vi "BT Tx Test Get Default LSL.vi"(8 "error in (no error)":errorcluster, 11 "Template Tx Test in":refnum<class "niDTS BT Tx Test.lvclass">) -> (0 "error out":errorcluster, 2 "Default LSL":T1 {"OBW Resutls"."Stop Frequency (Hz)" format="%#_4p"; "OBW Resutls"."Start Frequency (Hz)" format="%#_4p"}, 3 "Template Tx Test out":refnum<class "niDTS BT Tx Test.lvclass">)   [LabVIEW 2015, in "niDTS BT.lvlib" / "niDTS BT Tx Test.lvclass"]
uses:
  niDTS BT Tx Test.lvclass
  Includes/niDTS BT Tx Test INC Results.ctl
  Includes/niDTS BT Tx Test INC IBE Results.ctl
  Includes/niDTS BT Tx Test INC OBW Results.ctl
  Includes/niDTS BT Tx Test INC TXP Results.ctl
  Includes/niDTS BT Tx Test INC DEVM Results.ctl
  Includes/niDTS BT Tx Test INC CF Stability Results.ctl
  Includes/niDTS BT Tx Test INC CFO Resutls.ctl
  Includes/niDTS BT Tx Test INC Character Results.ctl
  niDTS BT Tx Test.lvclass/niDTS BT Tx Test.ctl
  Includes/niDTS BT Tx Test INC Default Limits.vi
  niDTS BT.lvlib
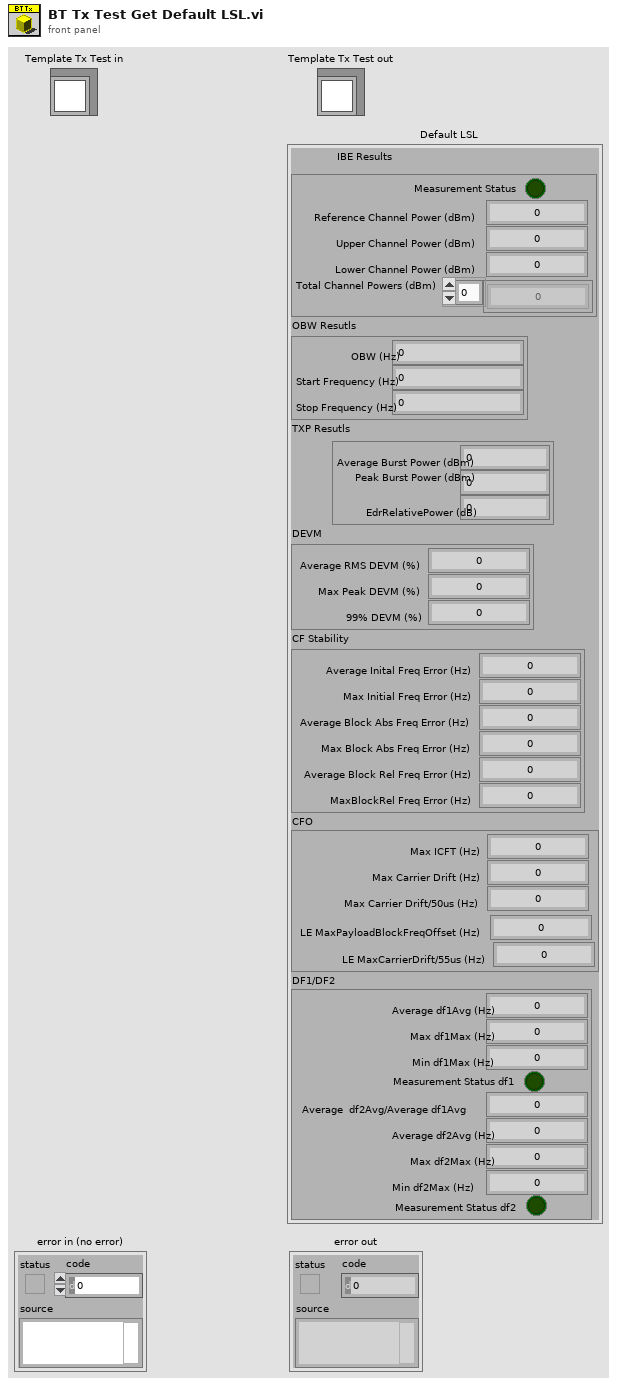
[diagram p1: front panel]
types:
  T1 = typedef "niDTS BT.lvlib/niDTS BT Tx Test INC Results.ctl" = cluster{"IBE Results":T2, "OBW Resutls":T3, "TXP Resutls":T4, "DEVM":T5, "CF Stability":T6, "CFO":T7, "DF1/DF2":T8}
  T2 = typedef "niDTS BT.lvlib/niDTS BT Tx Test INC IBE Results.ctl" = cluster{"Measurement Status":bool, "Reference Channel Power (dBm)":dbl, "Upper Channel Power (dBm)":dbl, "Lower Channel Power (dBm)":dbl, "Total Channel Powers (dBm)":dbl[]}
  T3 = typedef "niDTS BT.lvlib/niDTS BT Tx Test INC OBW Results.ctl" = cluster{"OBW (Hz)":dbl, "Start Frequency (Hz)":dbl, "Stop Frequency (Hz)":dbl}
  T4 = typedef "niDTS BT.lvlib/niDTS BT Tx Test INC TXP Results.ctl" = cluster{"Average Burst Power (dBm)":dbl, "Peak Burst Power (dBm)":dbl, "EdrRelativePower (dB)":dbl}
  T5 = typedef "niDTS BT.lvlib/niDTS BT Tx Test INC DEVM Results.ctl" = cluster{"Average RMS DEVM (%)":dbl, "Max Peak DEVM (%)":dbl, "99% DEVM (%)":dbl}
  T6 = typedef "niDTS BT.lvlib/niDTS BT Tx Test INC CF Stability Results.ctl" = cluster{"Average Inital Freq Error (Hz)":dbl, "Max Initial Freq Error (Hz)":dbl, "Average Block Abs Freq Error (Hz)":dbl, "Max Block Abs Freq Error (Hz)":dbl, "Average Block Rel Freq Error (Hz)":dbl, "MaxBlockRel Freq Error (Hz)":dbl}
  T7 = typedef "niDTS BT.lvlib/niDTS BT Tx Test INC CFO Resutls.ctl" = cluster{"Max ICFT (Hz)":dbl, "Max Carrier Drift (Hz)":dbl, "Max Carrier Drift/50us (Hz)":dbl, "LE MaxPayloadBlockFreqOffset (Hz)":dbl, "LE MaxCarrierDrift/55us (Hz)":dbl}
  T8 = typedef "niDTS BT.lvlib/niDTS BT Tx Test INC Character Results.ctl" = cluster{"Average df1Avg (Hz)":dbl, "Max df1Max (Hz)":dbl, "Min df1Max (Hz)":dbl, "Measurement Status df1":bool, "Average  df2Avg/Average df1Avg":dbl, "Average df2Avg (Hz)":dbl, "Max df2Max (Hz)":dbl, "Min df2Max (Hz)":dbl, "Measurement Status df2":bool}
  T9 = typedef "niDTS BT.lvlib/niDTS BT INC Packet Type.ctl" = enum16{"NULL", "POLL", "FHS", "DM1", "DH1", "HV1", "HV2", "HV3", "EV3", "DV", "AUX1", "DM3", "DH3", "EV4", "EV5", "DM5", "DH5", "LE-TP"}
  T10 = typedef "niDTS BT.lvlib/niDTS BT INC Standard.ctl" = enum16{"BDR", "EDR", "LE-TP"}
  T11 = typedef "niDTS BT.lvlib/niDTS BT Tx Test INC BD Payload Data.ctl" = enum16{"0", "1", "01", "00001111", "PN9", "AUTO"}
  T12 = typedef "niDTS BT.lvlib/niDTS BT Tx Test INC Modulation Characteristics.ctl" = enum16{"DF1", "DF2", "BOTH"}
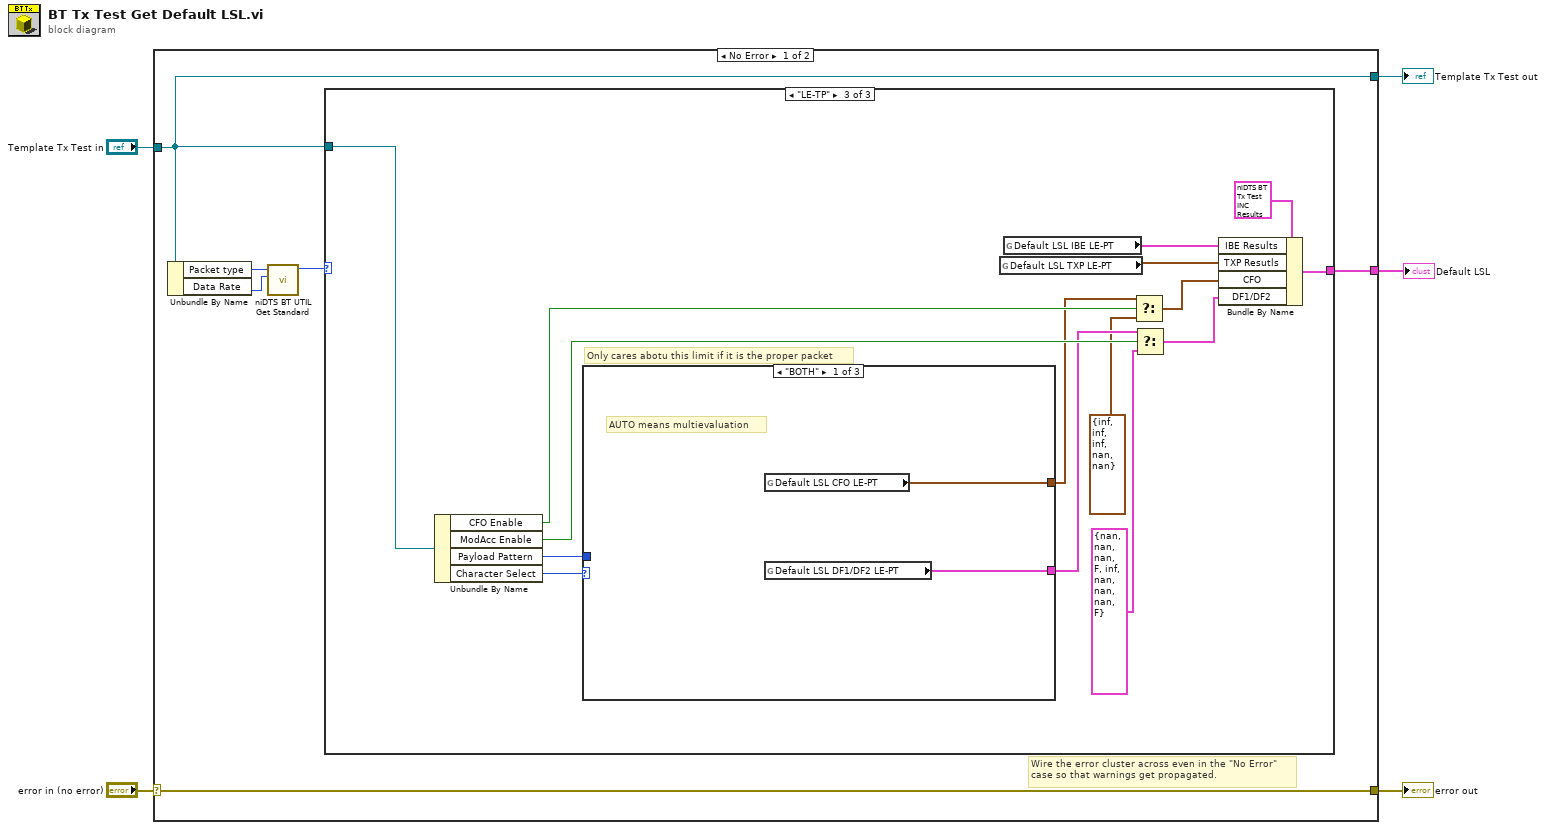
[diagram p0: block diagram]
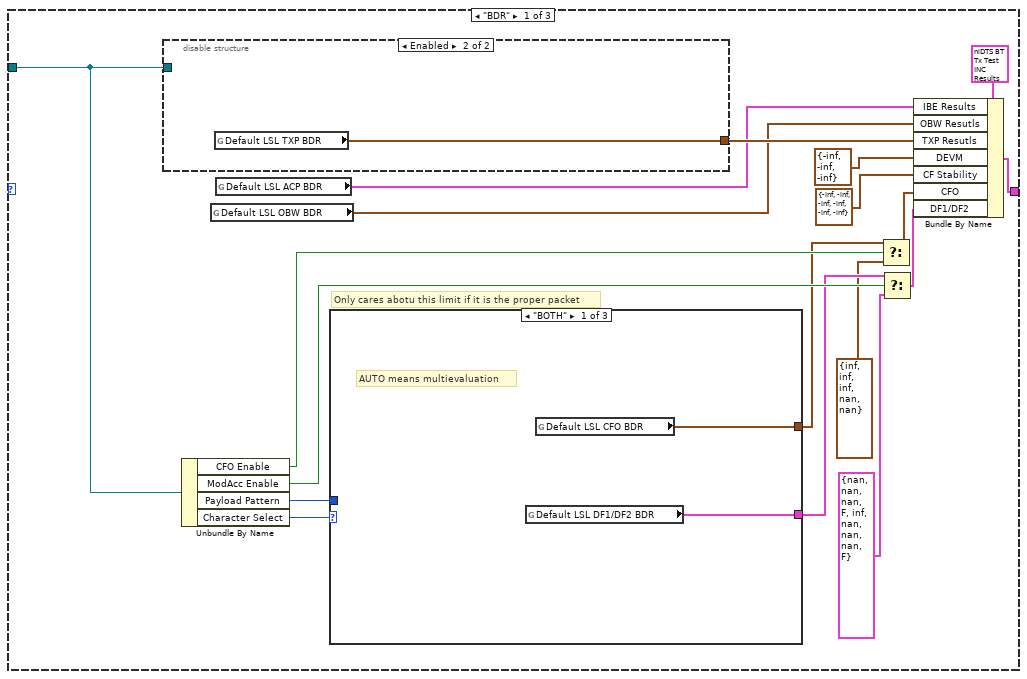
[diagram p2: hidden frame]
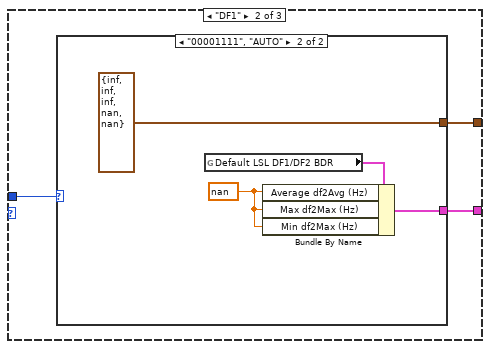
[diagram p3: hidden frame]
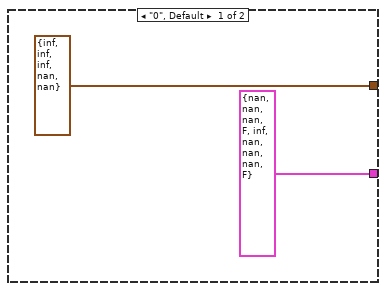
[diagram p4: hidden frame]
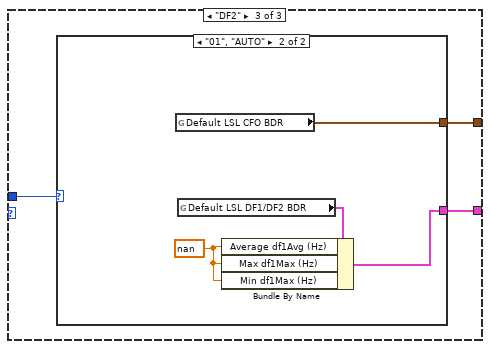
[diagram p5: hidden frame]
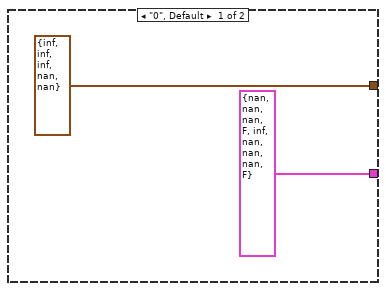
[diagram p6: hidden frame]
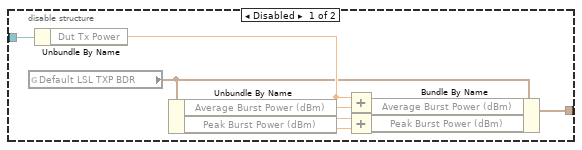
[diagram p7: hidden frame]
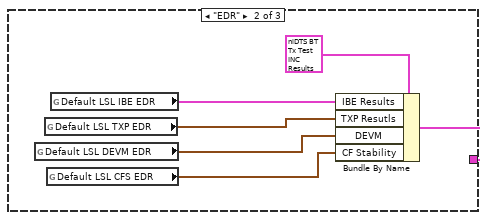
[diagram p8: hidden frame]
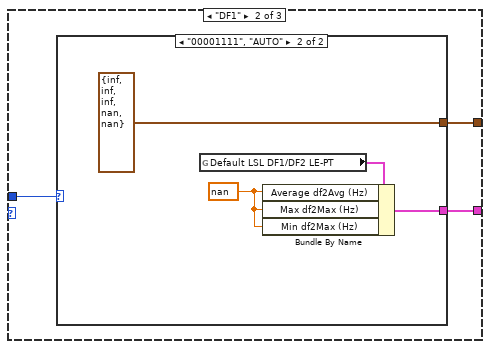
[diagram p9: hidden frame]
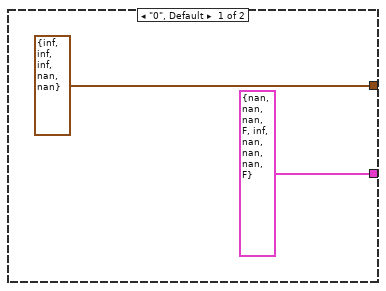
[diagram p10: hidden frame]
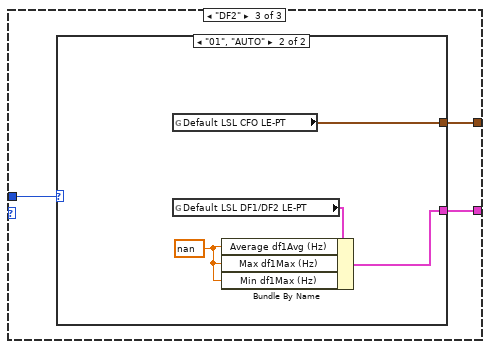
[diagram p11: hidden frame]
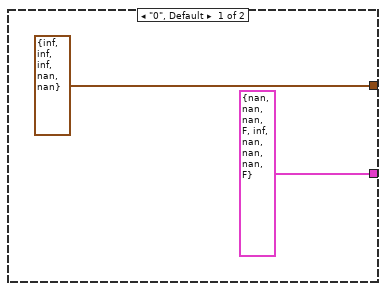
[diagram p12: hidden frame]
diagram:
  n1 = case shown="No Error" "error in (no error)" {
    selector: "error in (no error)" -> [w11 w101]
    tunnel: [w11 w101] -> w4
    tunnel: [w9 w100] -> w2
    tunnel: "Template Tx Test in" -> [w9 w100]
    tunnel: [w10 _] -> w1
    frame No Error {
      # "Wire the error cluster across even in the \"No Error\"\ncase so that warnings get propagated."
      n2 = Unbundle By Name(w9) -> ("Packet type"=w8:T9, "Data Rate"=w7:i32)
      n3 = call "niDTS BT UTIL Get Standard.vi"("Data Rate"=w7, "Packet type"=w8) -> ("BT Standard"=w6:T10)  [unwired: 9 in]
      n4 = case shown="\"LE-TP\"" w6 {
        tunnel: [w27 w59 w77] -> w10
        tunnel: w9 -> [w14 _ w67]
        frame "BDR" {
          # "Only cares abotu this limit if it is the proper packet"
          n5 = disable-structure shown="Enabled" {
            disable-tunnel: w14 -> [w57 _]
            disable-tunnel: [w51 w58] -> w28
            frame Disabled {
              n6 = global read "niDTS BT Tx Test INC Default Limits.vi" "Default LSL TXP BDR"() -> (w50:T4)
              n7 = Unbundle By Name(w57) -> ("Dut Tx Power"=w55:dbl)
              n8 = Unbundle By Name(w50) -> ("Average Burst Power (dBm)"=w56:dbl, "Peak Burst Power (dBm)"=w54:dbl)
              n9 = Add(x=w55, y=w56) -> (x+y=w53:dbl)
              n10 = Add(x=w55, y=w54) -> (x+y=w52:dbl)
              n11 = Bundle By Name(cluster=w50, "Average Burst Power (dBm)"=w53, "Peak Burst Power (dBm)"=w52) -> (w51:T4)
            }
            frame Enabled {
              n12 = global read "niDTS BT Tx Test INC Default Limits.vi" "Default LSL TXP BDR"() -> (w58:T4)
            }
          }
          n13 = Unbundle By Name(w14) -> ("CFO Enable"=w21:bool, "ModAcc Enable"=w20:bool, "Payload Pattern"=w22:T11, "Character Select"=w15:T12)
          n14 = global read "niDTS BT Tx Test INC Default Limits.vi" "Default LSL OBW BDR"() -> (w25:T3)
          n15 = global read "niDTS BT Tx Test INC Default Limits.vi" "Default LSL ACP BDR"() -> (w26:T2)
          n16 = case shown="\"BOTH\"" w15 {
            tunnel: [w30 w34 w43] -> w18
            tunnel: w22 -> [_ w33 w42]
            tunnel: [w31 w32 w41] -> w19
            frame "BOTH" {
              # "AUTO means multievaluation"
              n17 = global read "niDTS BT Tx Test INC Default Limits.vi" "Default LSL DF1/DF2 BDR"() -> (w30:T8)
              n18 = global read "niDTS BT Tx Test INC Default Limits.vi" "Default LSL CFO BDR"() -> (w31:T7)
            }
            frame "DF1" {
              n19 = case shown="\"00001111\", \"AUTO\"" w33 {
                tunnel: [T8 {"Average df1Avg (Hz)"=nan, "Max df1Max (Hz)"=nan, "Min df1Max (Hz)"=nan, "Measurement Status df1"=FALSE, "Average  df2Avg/Average df1Avg"=inf, "Average df2Avg (Hz)"=nan, "Max df2Max (Hz)"=nan, "Min df2Max (Hz)"=nan, "Measurement Status df2"=FALSE} ("Default USL DF1/DF2 BDR") w38] -> w34
                tunnel: [T7 {"Max ICFT (Hz)"=inf, "Max Carrier Drift (Hz)"=inf, "Max Carrier Drift/50us (Hz)"=inf, "LE MaxPayloadBlockFreqOffset (Hz)"=nan, "LE MaxCarrierDrift/55us (Hz)"=nan} ("f") T7 {"Max ICFT (Hz)"=inf, "Max Carrier Drift (Hz)"=inf, "Max Carrier Drift/50us (Hz)"=inf, "LE MaxPayloadBlockFreqOffset (Hz)"=nan, "LE MaxCarrierDrift/55us (Hz)"=nan} ("f")] -> w32
                frame "0", Default {
                }
                frame "00001111", "AUTO" {
                  w39 = nan ("Average df1Avg")
                  n20 = global read "niDTS BT Tx Test INC Default Limits.vi" "Default LSL DF1/DF2 BDR"() -> (w40:T8)
                  n21 = Bundle By Name(cluster=w40, "Average df2Avg (Hz)"=w39, "Max df2Max (Hz)"=w39, "Min df2Max (Hz)"=w39) -> (w38:T8)
                }
              }
            }
            frame "DF2" {
              n22 = case shown="\"01\", \"AUTO\"" w42 {
                tunnel: [T8 {"Average df1Avg (Hz)"=nan, "Max df1Max (Hz)"=nan, "Min df1Max (Hz)"=nan, "Measurement Status df1"=FALSE, "Average  df2Avg/Average df1Avg"=inf, "Average df2Avg (Hz)"=nan, "Max df2Max (Hz)"=nan, "Min df2Max (Hz)"=nan, "Measurement Status df2"=FALSE} ("Default USL DF1/DF2 BDR") w47] -> w43
                tunnel: [T7 {"Max ICFT (Hz)"=inf, "Max Carrier Drift (Hz)"=inf, "Max Carrier Drift/50us (Hz)"=inf, "LE MaxPayloadBlockFreqOffset (Hz)"=nan, "LE MaxCarrierDrift/55us (Hz)"=nan} ("f") w46] -> w41
                frame "0", Default {
                }
                frame "01", "AUTO" {
                  w48 = nan ("Average df1Avg")
                  n23 = global read "niDTS BT Tx Test INC Default Limits.vi" "Default LSL CFO BDR"() -> (w46:T7)
                  n24 = global read "niDTS BT Tx Test INC Default Limits.vi" "Default LSL DF1/DF2 BDR"() -> (w49:T8)
                  n25 = Bundle By Name(cluster=w49, "Average df1Avg (Hz)"=w48, "Max df1Max (Hz)"=w48, "Min df1Max (Hz)"=w48) -> (w47:T8)
                }
              }
            }
          }
          n26 = Select(t=w19, s=w21, f=T7 {"Max ICFT (Hz)"=inf, "Max Carrier Drift (Hz)"=inf, "Max Carrier Drift/50us (Hz)"=inf, "LE MaxPayloadBlockFreqOffset (Hz)"=nan, "LE MaxCarrierDrift/55us (Hz)"=nan}) -> (s? t:f=w13:T7)
          n27 = Select(t=w18, s=w20, f=T8 {"Average df1Avg (Hz)"=nan, "Max df1Max (Hz)"=nan, "Min df1Max (Hz)"=nan, "Measurement Status df1"=FALSE, "Average  df2Avg/Average df1Avg"=inf, "Average df2Avg (Hz)"=nan, "Max df2Max (Hz)"=nan, "Min df2Max (Hz)"=nan, "Measurement Status df2"=FALSE} ("Default USL DF1/DF2 BDR")) -> (s? t:f=w12:T8)
          n28 = Bundle By Name(cluster=T1 {"IBE Results"={"Measurement Status"=FALSE, "Reference Channel Power (dBm)"=0.0, "Upper Channel Power (dBm)"=0.0, "Lower Channel Power (dBm)"=0.0, "Total Channel Powers (dBm)"=[]}, "OBW Resutls"={"OBW (Hz)"=0.0, "Start Frequency (Hz)"=0.0, "Stop Frequency (Hz)"=0.0}, "TXP Resutls"={"Average Burst Power (dBm)"=-35.0, "Peak Burst Power (dBm)"=-35.0, "EdrRelativePower (dB)"=0.0}, "DEVM"={"Average RMS DEVM (%)"=0.0, "Max Peak DEVM (%)"=0.0, "99% DEVM (%)"=0.0}, "CF Stability"={"Average Inital Freq Error (Hz)"=0.0, "Max Initial Freq Error (Hz)"=0.0, "Average Block Abs Freq Error (Hz)"=0.0, "Max Block Abs Freq Error (Hz)"=0.0, "Average Block Rel Freq Error (Hz)"=0.0, "MaxBlockRel Freq Error (Hz)"=0.0}, "CFO"={"Max ICFT (Hz)"=0.0, "Max Carrier Drift (Hz)"=0.0, "Max Carrier Drift/50us (Hz)"=0.0, "LE MaxPayloadBlockFreqOffset (Hz)"=0.0, "LE MaxCarrierDrift/55us (Hz)"=0.0}, "DF1/DF2"={"Average df1Avg (Hz)"=0.0, "Max df1Max (Hz)"=0.0, "Min df1Max (Hz)"=0.0, "Measurement Status df1"=FALSE, "Average  df2Avg/Average df1Avg"=0.0, "Average df2Avg (Hz)"=0.0, "Max df2Max (Hz)"=0.0, "Min df2Max (Hz)"=0.0, "Measurement Status df2"=FALSE}} ("Default USL"), "IBE Results"=w26, "OBW Resutls"=w25, "TXP Resutls"=w28, "DEVM"=T5 {"Average RMS DEVM (%)"=-inf, "Max Peak DEVM (%)"=-inf, "99% DEVM (%)"=-inf}, "CF Stability"=T6 {"Average Inital Freq Error (Hz)"=-inf, "Max Initial Freq Error (Hz)"=-inf, "Average Block Abs Freq Error (Hz)"=-inf, "Max Block Abs Freq Error (Hz)"=-inf, "Average Block Rel Freq Error (Hz)"=-inf, "MaxBlockRel Freq Error (Hz)"=-inf}, "CFO"=w13, "DF1/DF2"=w12) -> (w27:T1)
        }
        frame "EDR" {
          n29 = global read "niDTS BT Tx Test INC Default Limits.vi" "Default LSL DEVM EDR"() -> (w61:T5)
          n30 = global read "niDTS BT Tx Test INC Default Limits.vi" "Default LSL TXP EDR"() -> (w60:T4)
          n31 = global read "niDTS BT Tx Test INC Default Limits.vi" "Default LSL CFS EDR"() -> (w62:T6)
          n32 = global read "niDTS BT Tx Test INC Default Limits.vi" "Default LSL IBE EDR"() -> (w63:T2)
          n33 = Bundle By Name(cluster=T1 {"IBE Results"={"Measurement Status"=FALSE, "Reference Channel Power (dBm)"=0.0, "Upper Channel Power (dBm)"=0.0, "Lower Channel Power (dBm)"=0.0, "Total Channel Powers (dBm)"=[]}, "OBW Resutls"={"OBW (Hz)"=0.0, "Start Frequency (Hz)"=0.0, "Stop Frequency (Hz)"=0.0}, "TXP Resutls"={"Average Burst Power (dBm)"=-35.0, "Peak Burst Power (dBm)"=-35.0, "EdrRelativePower (dB)"=0.0}, "DEVM"={"Average RMS DEVM (%)"=0.0, "Max Peak DEVM (%)"=0.0, "99% DEVM (%)"=0.0}, "CF Stability"={"Average Inital Freq Error (Hz)"=0.0, "Max Initial Freq Error (Hz)"=0.0, "Average Block Abs Freq Error (Hz)"=0.0, "Max Block Abs Freq Error (Hz)"=0.0, "Average Block Rel Freq Error (Hz)"=0.0, "MaxBlockRel Freq Error (Hz)"=0.0}, "CFO"={"Max ICFT (Hz)"=0.0, "Max Carrier Drift (Hz)"=0.0, "Max Carrier Drift/50us (Hz)"=0.0, "LE MaxPayloadBlockFreqOffset (Hz)"=0.0, "LE MaxCarrierDrift/55us (Hz)"=0.0}, "DF1/DF2"={"Average df1Avg (Hz)"=0.0, "Max df1Max (Hz)"=0.0, "Min df1Max (Hz)"=0.0, "Measurement Status df1"=FALSE, "Average  df2Avg/Average df1Avg"=0.0, "Average df2Avg (Hz)"=0.0, "Max df2Max (Hz)"=0.0, "Min df2Max (Hz)"=0.0, "Measurement Status df2"=FALSE}} ("Default USL"), "IBE Results"=w63, "TXP Resutls"=w60, "DEVM"=w61, "CF Stability"=w62) -> (w59:T1)
        }
        frame "LE-TP" {
          # "Only cares abotu this limit if it is the proper packet"
          n34 = Unbundle By Name(w67) -> ("CFO Enable"=w74:bool, "ModAcc Enable"=w73:bool, "Payload Pattern"=w75:T11, "Character Select"=w68:T12)
          n35 = case shown="\"BOTH\"" w68 {
            tunnel: [w80 w84 w93] -> w71
            tunnel: w75 -> [_ w83 w92]
            tunnel: [w81 w82 w91] -> w72
            frame "BOTH" {
              # "AUTO means multievaluation"
              n36 = global read "niDTS BT Tx Test INC Default Limits.vi" "Default LSL CFO LE-PT"() -> (w81:T7)
              n37 = global read "niDTS BT Tx Test INC Default Limits.vi" "Default LSL DF1/DF2 LE-PT"() -> (w80:T8)
            }
            frame "DF1" {
              n38 = case shown="\"00001111\", \"AUTO\"" w83 {
                tunnel: [T8 {"Average df1Avg (Hz)"=nan, "Max df1Max (Hz)"=nan, "Min df1Max (Hz)"=nan, "Measurement Status df1"=FALSE, "Average  df2Avg/Average df1Avg"=inf, "Average df2Avg (Hz)"=nan, "Max df2Max (Hz)"=nan, "Min df2Max (Hz)"=nan, "Measurement Status df2"=FALSE} ("Default USL DF1/DF2 BDR") w88] -> w84
                tunnel: [T7 {"Max ICFT (Hz)"=inf, "Max Carrier Drift (Hz)"=inf, "Max Carrier Drift/50us (Hz)"=inf, "LE MaxPayloadBlockFreqOffset (Hz)"=nan, "LE MaxCarrierDrift/55us (Hz)"=nan} ("f") T7 {"Max ICFT (Hz)"=inf, "Max Carrier Drift (Hz)"=inf, "Max Carrier Drift/50us (Hz)"=inf, "LE MaxPayloadBlockFreqOffset (Hz)"=nan, "LE MaxCarrierDrift/55us (Hz)"=nan} ("f")] -> w82
                frame "0", Default {
                }
                frame "00001111", "AUTO" {
                  w89 = nan ("Average df1Avg")
                  n39 = global read "niDTS BT Tx Test INC Default Limits.vi" "Default LSL DF1/DF2 LE-PT"() -> (w90:T8)
                  n40 = Bundle By Name(cluster=w90, "Average df2Avg (Hz)"=w89, "Max df2Max (Hz)"=w89, "Min df2Max (Hz)"=w89) -> (w88:T8)
                }
              }
            }
            frame "DF2" {
              n41 = case shown="\"01\", \"AUTO\"" w92 {
                tunnel: [T8 {"Average df1Avg (Hz)"=nan, "Max df1Max (Hz)"=nan, "Min df1Max (Hz)"=nan, "Measurement Status df1"=FALSE, "Average  df2Avg/Average df1Avg"=inf, "Average df2Avg (Hz)"=nan, "Max df2Max (Hz)"=nan, "Min df2Max (Hz)"=nan, "Measurement Status df2"=FALSE} ("Default USL DF1/DF2 BDR") w97] -> w93
                tunnel: [T7 {"Max ICFT (Hz)"=inf, "Max Carrier Drift (Hz)"=inf, "Max Carrier Drift/50us (Hz)"=inf, "LE MaxPayloadBlockFreqOffset (Hz)"=nan, "LE MaxCarrierDrift/55us (Hz)"=nan} ("f") w96] -> w91
                frame "0", Default {
                }
                frame "01", "AUTO" {
                  w98 = nan ("Average df1Avg")
                  n42 = global read "niDTS BT Tx Test INC Default Limits.vi" "Default LSL CFO LE-PT"() -> (w96:T7)
                  n43 = global read "niDTS BT Tx Test INC Default Limits.vi" "Default LSL DF1/DF2 LE-PT"() -> (w99:T8)
                  n44 = Bundle By Name(cluster=w99, "Average df1Avg (Hz)"=w98, "Max df1Max (Hz)"=w98, "Min df1Max (Hz)"=w98) -> (w97:T8)
                }
              }
            }
          }
          n45 = global read "niDTS BT Tx Test INC Default Limits.vi" "Default LSL TXP LE-PT"() -> (w76:T4)
          n46 = global read "niDTS BT Tx Test INC Default Limits.vi" "Default LSL IBE LE-PT"() -> (w78:T2)
          n47 = Select(t=w72, s=w74, f=T7 {"Max ICFT (Hz)"=inf, "Max Carrier Drift (Hz)"=inf, "Max Carrier Drift/50us (Hz)"=inf, "LE MaxPayloadBlockFreqOffset (Hz)"=nan, "LE MaxCarrierDrift/55us (Hz)"=nan}) -> (s? t:f=w65:T7)
          n48 = Select(t=w71, s=w73, f=T8 {"Average df1Avg (Hz)"=nan, "Max df1Max (Hz)"=nan, "Min df1Max (Hz)"=nan, "Measurement Status df1"=FALSE, "Average  df2Avg/Average df1Avg"=inf, "Average df2Avg (Hz)"=nan, "Max df2Max (Hz)"=nan, "Min df2Max (Hz)"=nan, "Measurement Status df2"=FALSE} ("Default USL DF1/DF2 BDR")) -> (s? t:f=w66:T8)
          n49 = Bundle By Name(cluster=T1 {"IBE Results"={"Measurement Status"=FALSE, "Reference Channel Power (dBm)"=0.0, "Upper Channel Power (dBm)"=0.0, "Lower Channel Power (dBm)"=0.0, "Total Channel Powers (dBm)"=[]}, "OBW Resutls"={"OBW (Hz)"=0.0, "Start Frequency (Hz)"=0.0, "Stop Frequency (Hz)"=0.0}, "TXP Resutls"={"Average Burst Power (dBm)"=-35.0, "Peak Burst Power (dBm)"=-35.0, "EdrRelativePower (dB)"=0.0}, "DEVM"={"Average RMS DEVM (%)"=0.0, "Max Peak DEVM (%)"=0.0, "99% DEVM (%)"=0.0}, "CF Stability"={"Average Inital Freq Error (Hz)"=0.0, "Max Initial Freq Error (Hz)"=0.0, "Average Block Abs Freq Error (Hz)"=0.0, "Max Block Abs Freq Error (Hz)"=0.0, "Average Block Rel Freq Error (Hz)"=0.0, "MaxBlockRel Freq Error (Hz)"=0.0}, "CFO"={"Max ICFT (Hz)"=0.0, "Max Carrier Drift (Hz)"=0.0, "Max Carrier Drift/50us (Hz)"=0.0, "LE MaxPayloadBlockFreqOffset (Hz)"=0.0, "LE MaxCarrierDrift/55us (Hz)"=0.0}, "DF1/DF2"={"Average df1Avg (Hz)"=0.0, "Max df1Max (Hz)"=0.0, "Min df1Max (Hz)"=0.0, "Measurement Status df1"=FALSE, "Average  df2Avg/Average df1Avg"=0.0, "Average df2Avg (Hz)"=0.0, "Max df2Max (Hz)"=0.0, "Min df2Max (Hz)"=0.0, "Measurement Status df2"=FALSE}} ("Default USL"), "IBE Results"=w78, "TXP Resutls"=w76, "CFO"=w65, "DF1/DF2"=w66) -> (w77:T1)
        }
      }
    }
    frame Error {
    }
  }
  "error out" <- w4
  "Template Tx Test out" <- w2
  "Default LSL" <- w1
